vi "Do.vi"(8 "error in (no error)":errorcluster, 10 "Actor in":refnum<class "Actor.lvclass">, 11 "Add Data with TS Msg":refnum<class "Add Data with TS Msg.lvclass">) -> (0 "error out":errorcluster, 2 "Actor out":refnum<class "Actor.lvclass">)   [LabVIEW 2018, in "BNT_XtGraph.lvlib" / "Add Data with TS Msg.lvclass"]
doc: "This VI delivers the message to the actor by calling the appropriate method(s) on the actor."
uses:
  Add Data with TS Msg.lvclass
  <vilib>/ActorFramework/Actor/Actor.lvclass
  BNT_XtGraph/BNT_XtGraph.lvclass
  C:/Program Files (x86)/National Instruments/LabVIEW 2018/vi.lib/ActorFramework/Actor/Actor.lvclass
  Add Data with TS Msg.lvclass/Add Data with TS Msg.ctl
  CSPP_Core/Messages/CSPP_AsyncCallbackMsg/CSPP_AsyncCallback Msg.lvclass
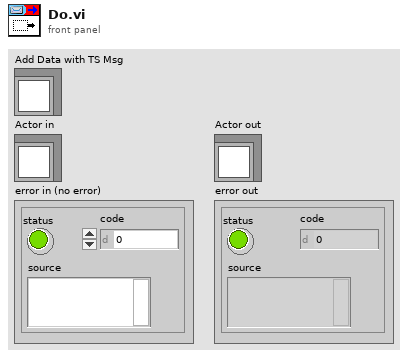
[diagram p1: front panel]
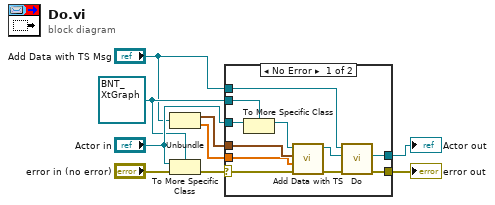
[diagram p0: block diagram]
diagram:
  w4 = refnum<class "BNT_XtGraph.lvclass"> refnum ("Actor in")
  n1 = Unbundle ("Main-Unbundler")("Add Data with TS Msg") -> (w2:timestamp, w1:dbl[])
  n2 = To More Specific Class(target class=w4, reference="Actor in", error in="error in (no error)") -> (error out=w8:errorcluster)  [unwired: 1 out]
  n3 = case shown="No Error" w8 {
    selector: w8 -> [w20 w22]
    tunnel: [w16 w22] -> w7
    tunnel: [w15 w21] -> w6
    tunnel: "Actor in" -> [w19 w21]
    tunnel: w4 -> [w18 _]
    tunnel: "Add Data with TS Msg" -> [w12 _]
    tunnel: w2 -> [w11 _]
    tunnel: w1 -> [w10 _]
    frame No Error {
      n4 = To More Specific Class ("To More Specific Class (internal)")(target class=w18, reference=w19) -> (specific class reference=w17:refnum<class "BNT_XtGraph.lvclass">)  [unwired: 1 in, 1 out]
      n5 = call "Add Data with TS.vi"("Error In"=w20, "Values"=w10, "Time Stamp"=w11, "BNT_XtGraph in"=w17) -> ("Error Out"=w13:errorcluster, "BNT_XtGraph out"=w14:refnum<class "BNT_XtGraph.lvclass">)  [unwired: 6 in]
      n6 = call-parent "Do.vi"("error in (no error)"=w13, "Actor in"=w14, "CSPP_AsyncCallback Msg"=w12) -> ("error out"=w16:errorcluster, "Actor out"=w15:refnum<class "Actor.lvclass">)  [unwired: 7 in]
    }
    frame Error {
    }
  }
  "error out" <- w7
  "Actor out" <- w6
